vi "TSC.vi"(0 "参数":string[](array[string])=["123456789123456", "", "", "10000", "", "", "21214", "", "512", "PASS"]) -> ()   [LabVIEW 2020]
uses:
  <vilib>/Utility/NIReport.llb/Report Type.ctl
  <vilib>/Utility/NIReport.llb/NI_report.lvclass
  <vilib>/Utility/NIReport.llb/NI_ReportGenerationCore.lvlib
  <vilib>/Utility/NIReport.llb/Excel/NI_Excel.lvclass
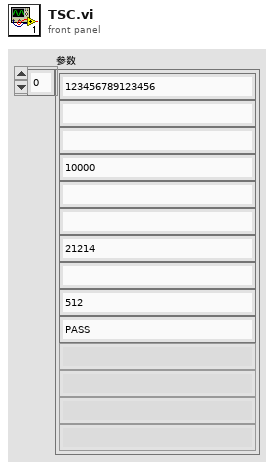
[diagram p1: front panel]
types:
  T1 = typedef "NI_ReportGenerationCore.lvlib/Report Type.ctl" = enum16{"HTML", "Word", "Excel"}
  T2 = enum16{"maximized", "minimized", "normal", "no change"}
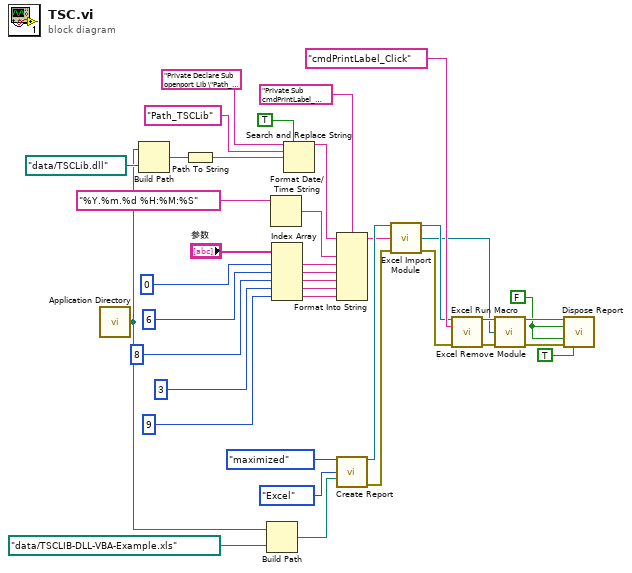
[diagram p0: block diagram]
diagram:
  w21 = FALSE ("wait until printing completed? (T)")
  n1 = call <vilib>:"Application Directory.vi"() -> ("Application Directory"=w18:path)
  n2 = Build Path(base path=w18, name or relative path=path "data/TSCLib.dll") -> (appended path=w22:path)
  n3 = Path To String(path=w22) -> (string=w25:string)
  n4 = Build Path(base path=w18, name or relative path=path "data/TSCLIB-DLL-VBA-Example.xls" ("template (empty)")) -> (appended path=w19:path)
  n5 = Format Date/Time String(time format string (%c)="%Y.%m.%d %H:%M:%S") -> (date/time string=w16:string)  [unwired: 2 in]
  n6 = Index Array(array="参数", index #1=0 ("index"), index #2=6 ("index"), index #3=8 ("index"), index #4=3 ("index"), index #5=9 ("index")) -> (element #1=w9:string, element #2=w6:string, element #3=w5:string, element #4=w3:string, element #5=w1:string)
  n7 = Search and Replace String(replace all?=TRUE ("replace all? (F)"), input string="Private Declare Sub openport Lib \"Path_TSCLib\" (ByVal PrinterName As String)\nPrivate Declare Sub closeport Lib \"Path_TSCLib\" ()\nPrivate Declare Sub sendcommand Lib \"Path_TSCLib\" (ByVal command As String)\nPrivate Declare Sub setup Lib \"Path_TSCLib\" ( _\n        ByVal LabelWidth As String, _\n        ByVal LabelHeight As String, _\n        ByVal Speed As String, _\n        ByVal Density As String, _\n        ByVal Sensor As String, _\n        ByVal Vertical As String, _\n        ByVal Offset As String)\nPrivate Declare Sub downloadpcx Lib \"Path_TSCLib\" ( _\n        ByVal Filename As String, _\n        ByVal ImageName As String)\nPrivate Declare Sub barcode Lib \"Path_TSCLib\" ( _\n        ByVal X As String, _\n    ByVal Y As String, _\n    ByVal CodeType As String, _\n    ByVal Height As String, _\n    ByVal Readable As String, _\n    ByVal rotation As String, _\n    ByVal Narrow As String, _\n    ByVal Wide As String, _\n    ByVal Code As String)\nPrivate Declare Sub printerfont Lib \"Path_TSCLib\" ( _\n    ByVal X As String, _\n    ByVal Y As String, _\n    ByVal FontName As String, _\n    ByVal rotation As String, _\n    ByVal Xmul As String, _\n    ByVal Ymul As String, _\n    ByVal Content As String)\nPrivate Declare Sub clearbuffer Lib \"Path_TSCLib\" ()\nPrivate Declare Sub printlabel Lib \"Path_TSCLib\" ( _\n    ByVal NumberOfSet As String, _\n    ByVal NumberOfCopy As String)\nPrivate Declare Sub formfeed Lib \"Path_TSCLib\" ()\nPrivate Declare Sub nobackfeed Lib \"Path_TSCLib\" ()\nPrivate Declare Sub windowsfont Lib \"Path_TSCLib\" ( _\n    ByVal X As Integer, _\n    ByVal Y As Integer, _\n    ByVal fontheight As Integer, _\n    ByVal rotation As Integer, _\n    ByVal fontstyle As Integer, _\n    ByVal fontunderline As Integer, _\n    ByVal FaceName As String, _\n    ByVal TextContent As String)\n\nPrivate Declare Sub windowsfontU Lib \"Path_TSCLib\" ( _\n    ByVal X As Integer, _\n    ByVal Y As Integer, _\n    ByVal fontheight As Integer, _\n    ByVal rotation As Integer, _\n    ByVal fontstyle As Integer, _\n    ByVal fontunderline As Integer, _\n    ByVal FaceName As String, _\n    ByVal TextContent As String)\n\nPrivate Declare Sub about Lib \"Path_TSCLib\" ()\n\nPrivate Declare Function isusbportready Lib \"Path_TSCLib\" () As Integer\nPrivate Declare Function usbportqueryprinter Lib \"Path_TSCLib\" () As Integer\nPrivate Declare Function usbportwrite Lib \"Path_TSCLib\" (ByVal command As String) As Integer\n\n" ("module code (\"\")"), search string="Path_TSCLib", replace string=w25) -> (result string=w14:string)  [unwired: 4 in, 3 out]
  n8 = Format Into String(format string="Private Sub cmdPrintLabel_Click()\n    Call openport(\"TSC TTP-244 Pro\")\n    Call setup(\"101.6\", \"39.54\", \"5\", \"11\", \"0\", \"3\", \"0\")\n    Call clearbuffer\n    Call sendcommand(\"DIRECTION 1\")\n    'Call windowsfont(180, 0, 8, 0, 0, 1, \"宋体\", \"————————————————————————————————————————————————————————\")\n    Call windowsfont(305, 10, 35, 0, 0, 0, \"宋体\", \"水冷气密测试\")\n    'Call windowsfont(180, 50, 8, 0, 0, 1, \"宋体\", \"————————————————————————————————————————————————————————\")\n    Call windowsfont(180, 60, 30, 0, 0, 0, \"宋体\", \"测试时间：\" + \"%s\")\n    'Call windowsfont(180, 95, 8, 0, 0, 1, \"宋体\", \"————————————————————————————————————————————————————————\")\n    Call windowsfont(180, 100, 30, 0, 0, 0, \"宋体\", \"PACK编码：\" + \"%s\")\n    'Call windowsfont(180, 135, 8, 0, 0, 1, \"宋体\", \"————————————————————————————————————————————————————————\")\n    Call windowsfont(180, 140, 30, 0, 0, 0, \"宋体\", \"保持压力值(Pa)：\" + \"%s\")\n   ' Call windowsfont(180, 175, 8, 0, 0, 1, \"宋体\", \"————————————————————————————————————————————————————————\")\n    Call windowsfont(180, 180, 30, 0, 0, 0, \"宋体\", \"测试总时间(s)：\" + \"%s\")\n   ' Call windowsfont(180, 215, 8, 0, 0, 1, \"宋体\", \"————————————————————————————————————————————————————————\")\n    Call windowsfont(180, 220, 30, 0, 0, 0, \"宋体\", \"泄漏值(Pa)：\" + \"%s\")\n    'Call windowsfont(180, 255, 8, 0, 0, 1, \"宋体\", \"————————————————————————————————————————————————————————\")\n    Call windowsfont(180, 260, 30, 0, 0, 0, \"宋体\", \"测试结果：\" + \"%s\")\n   ' Call windowsfont(180, 285, 8, 0, 0, 1, \"宋体\", \"————————————————————————————————————————————————————————\")\n    'Call barcode(\"200\", \"200\", \"128\", \"100\", \"1\", \"0\", \"2\", \"2\", txtBarcodeValue.Text)\n    Call sendcommand(\"SET CUTTER 1\")\n    Call printlabel(\"1\", \"1\")\n    Call closeport\nEnd Sub\n" ("module code (\"\")"), initial string=w14, w16, w9, w6, w5, w3, w1) -> (resulting string=w17:string)  [unwired: 1 in, 1 out]
  n9 = call <vilib>:"Create Report.vi"("window state (normal)"=T2."maximized", "report type"=Report_Type."Excel", "template (empty)"=w19) -> ("report out"=w34:refnum<class "NI_report.lvclass">, "error out"=w35:errorcluster)  [unwired: 11 in]
  n10 = call <vilib>:"Excel Import Module.vi"("report in"=w34, "module code (\"\")"=w17, "error in (no error)"=w35) -> ("report out"=w33:refnum<class "NI_report.lvclass">, "module reference"=w24:refnum<k7>, "error out"=w32:errorcluster)  [unwired: 10 in]
  n11 = call <vilib>:"Excel Run Macro.vi"("report in"=w33, "macro name"="cmdPrintLabel_Click", "error in (no error)"=w32) -> ("report out"=w31:refnum<class "NI_report.lvclass">, "error out"=w30:errorcluster)  [unwired: 10 in, 1 out]
  n12 = call <vilib>:"Excel Remove Module.vi"("report in"=w31, "module reference"=w24, "error in (no error)"=w30) -> ("report out"=w29:refnum<class "NI_report.lvclass">, "error out"=w28:errorcluster)  [unwired: 11 in]
  n13 = call-dynamic "Dispose Report.vi"("report in"=w29, "wait until printing completed? (T)"=w21, "save changes? (F)"=w21, "error in (no error)"=w28, "close report? (T)"=TRUE ("wait until printing completed? (T)")) -> ()  [unwired: 10 in, 1 out]
